vi "GetBinnedData.vi"(0 "VISA resource name":refnum<visa-resource-name>, 1 "Show on call?":bool=TRUE, 3 "Maximum Value":dbl=nan format="%#_13g", 5 "Time in ms (30000)":u32=30000, 9 "Time between calibrations (ms)":u32=1000, 11 "error in":errorcluster, 12 "# bins":i32=100, 14 "Minimum Value":dbl=nan format="%#_13g") -> (4 "VISA resource name out":refnum<visa-resource-name>, 6 "Binned time":dbl[](array[numeric]), 10 "Unbinned times / s":dbl[](array[numeric]), 15 "error out":errorcluster)   [LabVIEW 2017, in "GP22_TDC_Arduinoed.lvlib"]
doc: "Get data in the format that the ORTEC used to output. \n\nThis VI will take measurements for a given amount of time, bin the timings and output an array of the binned data."
uses:
  GP22_TDC_Arduinoed.lvlib
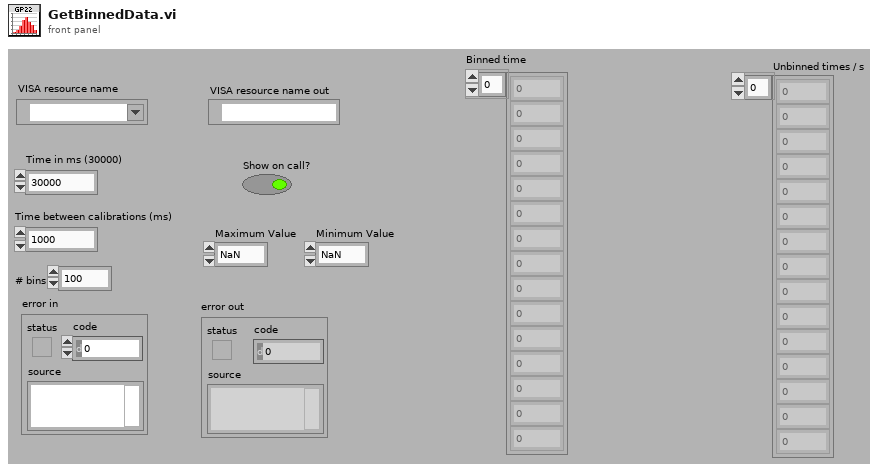
[diagram p1: front panel]
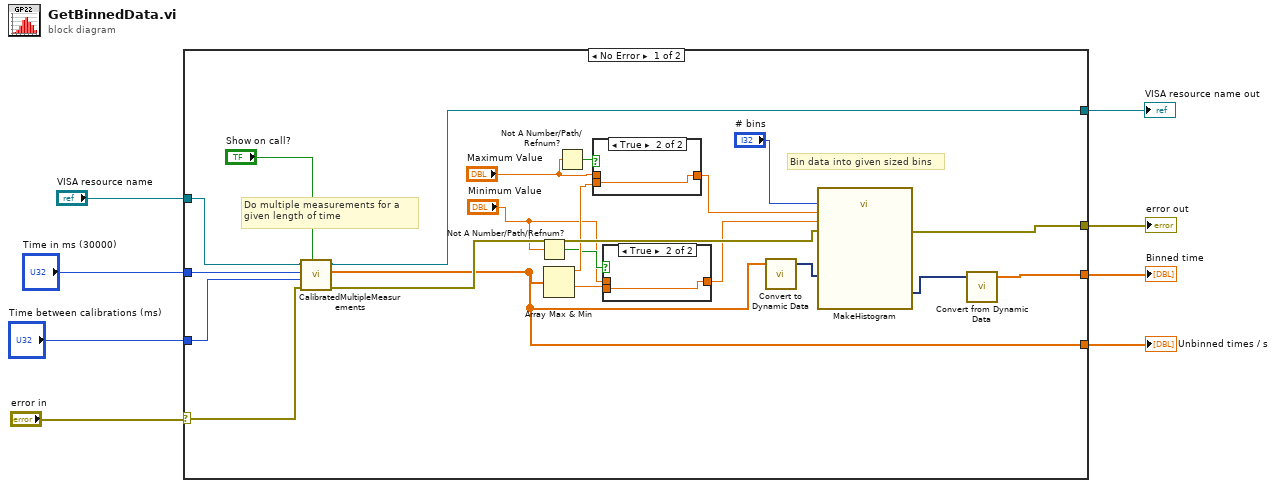
[diagram p0: block diagram]
diagram:
  n1 = case shown="No Error" "error in" {
    selector: "error in" -> [w18 w35]
    tunnel: "VISA resource name" -> [w29 w34]
    tunnel: "Time in ms (30000)" -> [w28 _]
    tunnel: [w27 w34] -> w6
    tunnel: "Time between calibrations (ms)" -> [w25 _]
    tunnel: [w14 _] -> w4
    tunnel: [w22 w35] -> w3
    tunnel: [w19 _] -> w2
    frame No Error {
      # "Bin data into given sized bins"
      # "Do multiple measurements for a \ngiven length of time"
      n2 = call "CalibratedMultipleMeasurements.vi"("Show on call?"="Show on call?", "error in"=w18, "Time between calibrations (ms)"=w25, "Time / ms (30000)"=w28, "VISA resource name"=w29) -> ("error out"=w23:errorcluster, "Times / s"=w14:dbl[], "VISA resource name out"=w27:refnum<visa-resource-name>)  [unwired: 3 in, 1 out]
      n3 = Not A Number/Path/Refnum?(number/path/refnum="Minimum Value") -> (NaN/Path/Refnum?=w11:bool)
      n4 = Array Max & Min(array=w14) -> (max value=w13:dbl, min value=w12:dbl)  [unwired: 2 out]
      n5 = Not A Number/Path/Refnum?(number/path/refnum="Maximum Value") -> (NaN/Path/Refnum?=w17:bool)
      n6 = case shown="True" w17 {
        tunnel: [w32 w33] -> w16
        tunnel: "Maximum Value" -> [w32 _]
        tunnel: w13 -> [_ w33]
        frame False {
        }
        frame True {
        }
      }
      n7 = case shown="True" w11 {
        tunnel: [w30 w31] -> w9
        tunnel: "Minimum Value" -> [w30 _]
        tunnel: w12 -> [_ w31]
        frame False {
        }
        frame True {
        }
      }
      n8 = call "Convert to Dynamic Data"("Array"=w14) -> ("Dynamic Data Type"=w24:dynamicdata)  [unwired: 3 in]
      n9 = call "MakeHistogram.vi"("Signal"=w24, "Number of Bins"="# bins", "Maximum Value"=w16, "Minimum Value"=w9, "error in (no error)"=w23) -> ("Histogram"=w20:dynamicdata, "error out"=w22:errorcluster)  [unwired: 9 in]
      n10 = call "Convert from Dynamic Data"("Dynamic Data Type"=w20) -> ("Array"=w19:dbl[])  [unwired: 3 in]
    }
    frame Error {
    }
  }
  "VISA resource name out" <- w6
  "error out" <- w3
  "Binned time" <- w2
  "Unbinned times / s" <- w4
